vi "SIM Runge-Kutta embedded Eval Err.vi"(0 "outputs":dbl[](array[numeric]), 1 "step accepted?":bool, 2 "step size":dbl, 3 "proposed step size":dbl, 4 "min step size":dbl, 5 "max step size":dbl, 6 "error order":i32, 7 "max step ratio":dbl, 8 "error coefficients":dbl[](array[numeric]), 9 "min float":dbl, 10 "k sub i":dbl[][](array[numeric]), 11 "relative tolerance":dbl, 12 "Zero Array":dbl[](array[numeric]), 13 "absolute tolerance":dbl) -> (14 "k sub i out":dbl[][](array[numeric]), 15 "Zero Array Out":dbl[](array[numeric]), 16 "outputs out":dbl[](array[numeric]), 17 "proposed step size out":dbl, 18 "new step size ratio":dbl, 19 "step accepted? out":bool)   [LabVIEW 2020]
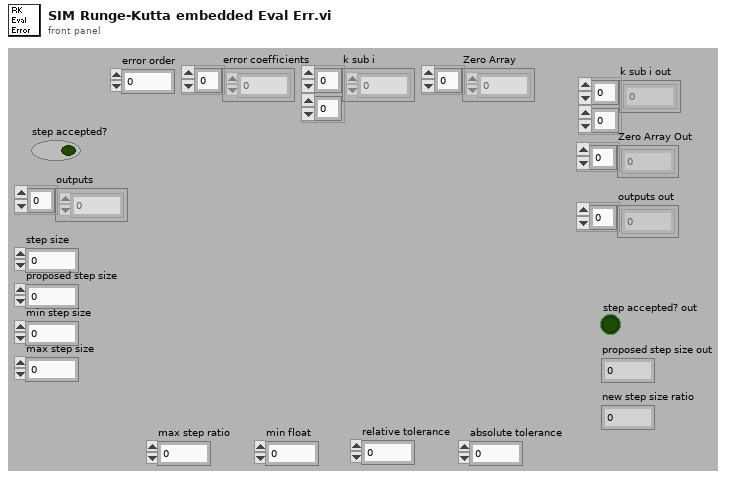
[diagram p1: front panel]
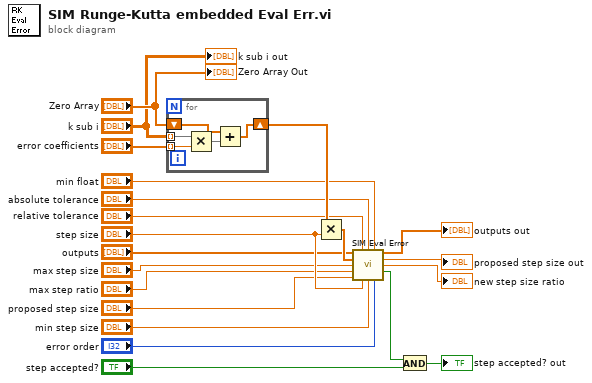
[diagram p0: block diagram]
diagram:
  n1 = for {
    tunnel: "k sub i" -> [w26] mode=indexing
    tunnel: "error coefficients" -> [w25] mode=indexing
    shift-right: [w23] -> w20
    shift-left: "Zero Array" -> [w22]
    n2 = Multiply(x=w26, y=w25) -> (x*y=w24:dbl[])
    n3 = Add(x=w22, y=w24) -> (x+y=w23:dbl[])
  }
  n4 = Multiply(x=w20, y="step size") -> (x*y=w15:dbl[])
  n5 = call "SIM Eval Error.vi"("Solution"="outputs", "relative tolerance"="relative tolerance", "absolute tolerance"="absolute tolerance", "min float"="min float", "estimated error"=w15, "max step size"="max step size", "max step ratio"="max step ratio", "proposed step size"="proposed step size", "step size"="step size", "min step size"="min step size", "error order"="error order") -> ("Solution Out"=→"outputs out":dbl[], "proposed step size out"=→"proposed step size out":dbl, "new step size ratio"=→"new step size ratio":dbl, "step accepted?"=w3:bool)  [unwired: 1 out]
  n6 = And(x=w3, y="step accepted?") -> (x .and. y?=→"step accepted? out":bool)
  "k sub i out" <- "k sub i"
  "Zero Array Out" <- "Zero Array"
